vi "mod_AM DSB CE Modulation.vi"(7 "carrier phase [rad]":dbl format="%.2f", 8 "ka":dbl format="%.2f", 11 "x":dbl[](array[numeric]) format="%.2f") -> (3 "AM DSB CE":cdb[](array[numeric]) format="%.2f")   [LabVIEW 2020, in "niAMT.lvlib"]
doc: "This VI performs double side band AM modulation with carrier. The output of this VI is the base band complex envelope of the modulated signal."
uses:
  <vilib>/addons/Modulation/niAMT.lvlib
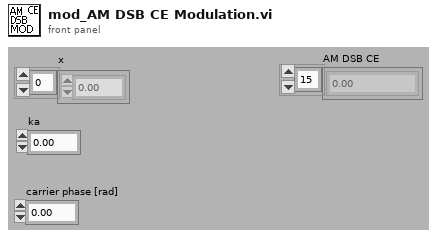
[diagram p1: front panel]
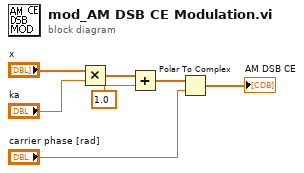
[diagram p0: block diagram]
diagram:
  n1 = Multiply(x="x", y="ka") -> (x*y=w5:dbl[])
  n2 = Add(x=w5, y=1.0) -> (x+y=w2:dbl[])
  n3 = Polar To Complex(1:"carrier phase [rad]", 2:w2) -> (0:→"AM DSB CE":cdb[])
